vi "Mak Cash Estimator.vi"(10 "Update Stats File?":bool=TRUE, 11 "file path (use dialog)":path=path "C:/Users/manma/Google Drive/WPC Stat Scrape/Data/WPC Stats.bin") -> (0 "Full WPC Stats":T1[][](array[typedef]) {"Date Updated" format="%<%m/%d/%Y>T"}, 1 "Profit/Day":dbl, 2 "Current Value":dbl format="%#_8g", 3 "Cash Profit Over Time":cluster{timestamp[], "Best Linear Fit":dbl[]}[](graph))   [LabVIEW 2021]
uses:
  SubVIs/WPC Player and Financial Stats.ctl
  <vilib>/Analysis/NI_AALPro.lvlib
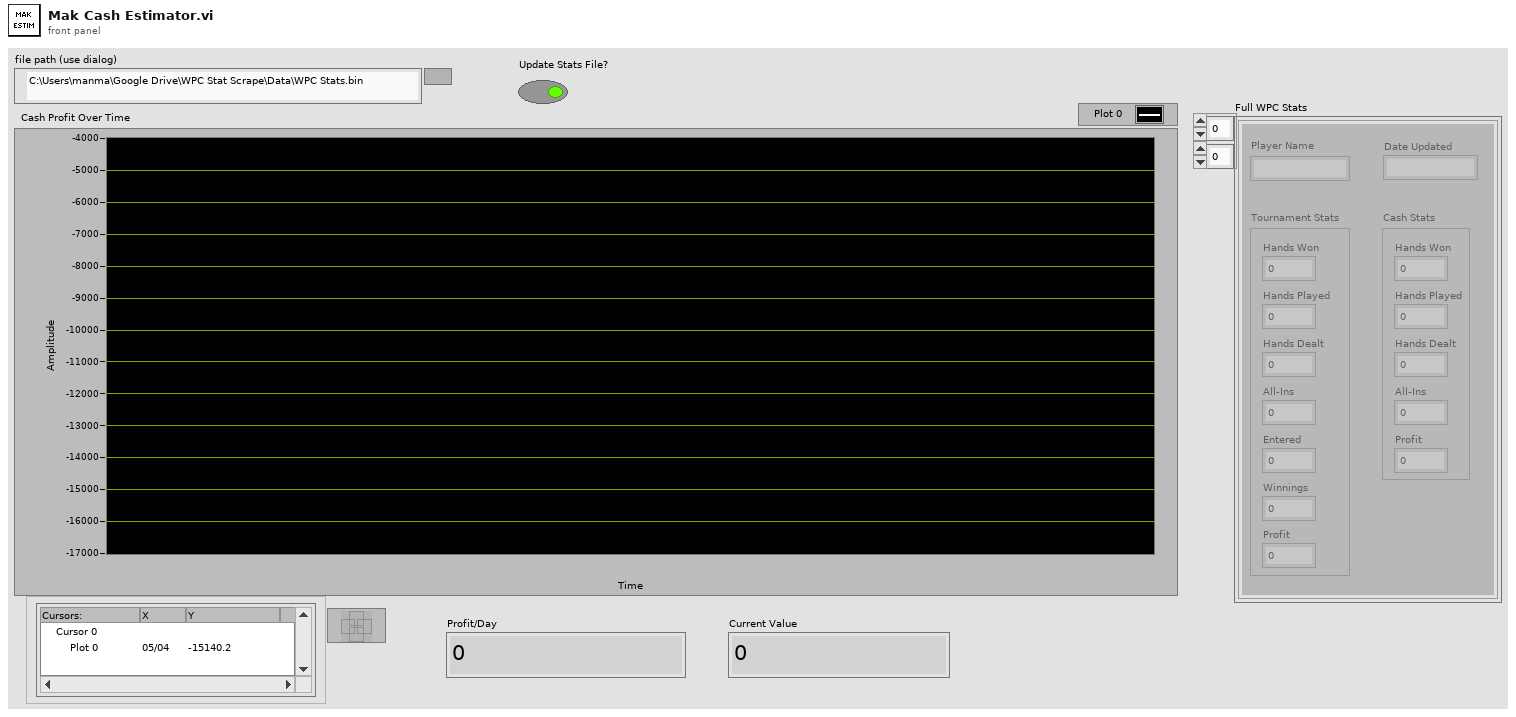
[diagram p1: front panel]
types:
  T1 = typedef "WPC Player and Financial Stats.ctl" = cluster{"Player Name":string, "Date Updated":timestamp, "Tournament Stats":cluster{"Hands Won":i32, "Hands Played":i32, "Hands Dealt":i32, "All-Ins":i32, "Entered":i32, "Winnings":dbl, "Profit":dbl}, "Cash Stats":cluster{"Hands Won":i32, "Hands Played":i32, "Hands Dealt":i32, "All-Ins":i32, "Profit":dbl}}
  T2 = typedef "LVDateTimeRec.ctl" = cluster{"fractional second":dbl, "second":i32, "minute":i32, "hour":i32, "day of month":i32, "month":i32, "year":i32, "day of week":i32, "day of year":i32, "DST":i32}
  T3 = enum16{"open", "replace", "create", "open or create", "replace or create", "replace or create with confirmation"}
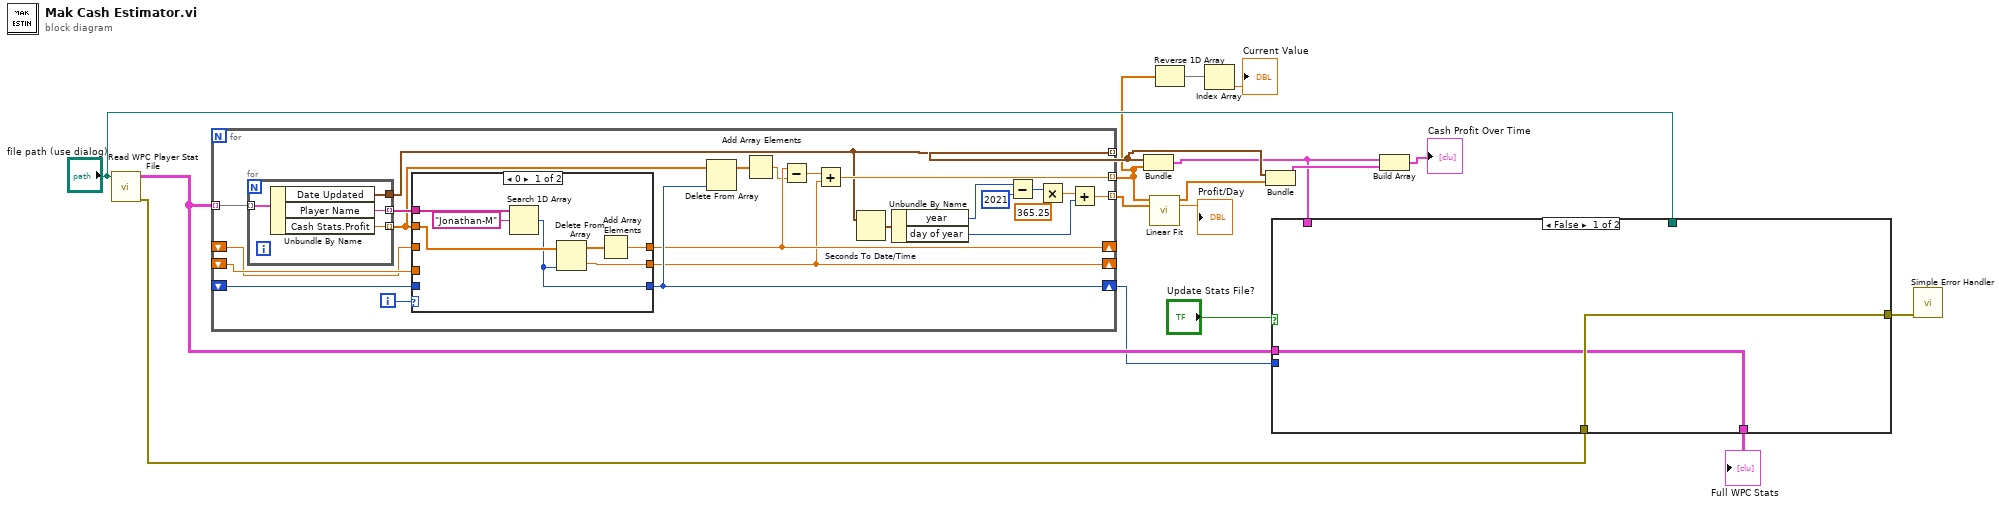
[diagram p0: block diagram]
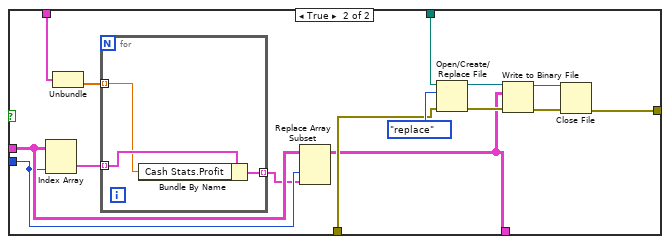
[diagram p2: hidden frame]
diagram:
  n1 = call "Read WPC Player Stat File.vi"("file path (use dialog)"="file path (use dialog)") -> ("error out"=w8:errorcluster, "Full WPC Stats"=w11:T1[][])  [unwired: 8 in, 1 out]
  n2 = for {
    tunnel: w11 -> [w40] mode=indexing
    shift-right: [w29] -> _
    shift-left: _ -> [w35]
    shift-right: [w27] -> _
    shift-left: _ -> [w36]
    shift-right: [w33] -> w10
    shift-left: _ -> [w37]
    tunnel: [w30] -> w4 mode=indexing
    tunnel: [w26] -> w15 mode=indexing
    tunnel: [w18] -> w5 mode=indexing
    i -> [w39]
    n3 = for {
      tunnel: w40 -> [w54] mode=indexing
      tunnel: [w53] -> w26
      tunnel: [w52] -> w38 mode=indexing
      tunnel: [w51] -> w34 mode=indexing
      n4 = Unbundle By Name(w54) -> ("Date Updated"=w53:timestamp, "Player Name"=w52:string, "Cash Stats.Profit"=w51:dbl)
    }
    n5 = case shown="0" w39 {
      tunnel: w38 -> [w47 _]
      tunnel: w34 -> [w45 _]
      tunnel: [w43 w48] -> w29
      tunnel: [w42 w49] -> w27
      tunnel: [w41 w50] -> w33
      tunnel: w37 -> [_ w50]
      tunnel: w36 -> [_ w49]
      tunnel: w35 -> [_ w48]
      frame 0 {
        n6 = Search 1D Array(1D array=w47, element="Jonathan-M") -> (index of element=w41:i32)  [unwired: 1 in]
        n7 = Delete From Array(array=w45, index=w41) -> (deleted portion=w42:dbl, array with subset deleted=w44:dbl[])  [unwired: 1 in]
        n8 = Add Array Elements(numeric array=w44) -> (sum=w43:dbl)
      }
      frame 1.., Default {
      }
    }
    n9 = Delete From Array(array=w34, index=w33) -> (array with subset deleted=w32:dbl[])  [unwired: 1 in, 1 out]
    n10 = Add Array Elements(numeric array=w32) -> (sum=w28:dbl)
    n11 = Subtract(x=w29, y=w28) -> (x-y=w31:dbl)
    n12 = Add(x=w31, y=w27) -> (x+y=w30:dbl)
    n13 = Seconds To Date/Time(time stamp (now)=w26) -> (date time rec=w25:T2)  [unwired: 1 in]
    n14 = Unbundle By Name(w25) -> ("year"=w24:i32, "day of year"=w19:i32)
    n15 = Subtract(x=w24, y=2021) -> (x-y=w22:i32)
    n16 = Multiply(x=w22, y=sgl 365.25) -> (x*y=w20:sgl)
    n17 = Add(x=w20, y=w19) -> (x+y=w18:sgl)
  }
  n18 = Bundle(w15, w4) -> (w9:cluster{timestamp[], dbl[]})  [unwired: 1 in]
  n19 = call <vilib>:"Linear Fit.vi"("Y"=w4, "X"=w5) -> ("Best Linear Fit"=w14:dbl[], "slope"=→"Profit/Day":dbl)  [unwired: 9 in, 3 out]
  n20 = Reverse 1D Array(array=w4) -> (reversed array=w3:dbl[])
  n21 = Index Array(array=w3) -> (element=→"Current Value":dbl)  [unwired: 1 in]
  n22 = Bundle(w15, "Best Linear Fit"=w14) -> (w16:cluster{timestamp[], "Best Linear Fit":dbl[]})  [unwired: 1 in]
  n23 = case shown="False" "Update Stats File?" {
    tunnel: w11 -> [w55 w68]
    tunnel: w10 -> [_ w67]
    tunnel: w9 -> [_ w71]
    tunnel: w8 -> [w56 w60]
    tunnel: "file path (use dialog)" -> [_ w59]
    tunnel: [w56 w58] -> w6
    tunnel: [w55 w57] -> w1
    frame False {
    }
    frame True {
      n24 = Index Array(array=w68, index (col)=w67) -> (element=w70:T1[])  [unwired: 1 in]
      n25 = Unbundle(w71) -> (w69:dbl[])  [unwired: 1 out]
      n26 = for {
        tunnel: w70 -> [w74] mode=indexing
        tunnel: w69 -> [w73] mode=indexing
        tunnel: [w72] -> w66 mode=indexing
        n27 = Bundle By Name(cluster=w74, "Cash Stats.Profit"=w73) -> (w72:T1)
      }
      n28 = Replace Array Subset(array=w68, new element=w66, index (col)=w67) -> (w57:T1[][])  [unwired: 1 in]
      n29 = Open/Create/Replace File(file path (use dialog)=w59, error in=w60, operation (0:open)=T3."replace") -> (refnum out=w63:refnum<file>, error out=w64:errorcluster)  [unwired: 3 in, 1 out]
      n30 = Write to Binary File(file (use dialog)=w63, data=w57, error in=w64) -> (refnum out=w62:refnum<file>, error out=w61:errorcluster)  [unwired: 3 in, 1 out]
      n31 = Close File(refnum=w62, error in=w61) -> (error out=w58:errorcluster)  [unwired: 1 out]
    }
  }
  "Full WPC Stats" <- w1
  n32 = Build Array(w9, w16) -> (→"Cash Profit Over Time":cluster{timestamp[], "Best Linear Fit":dbl[]}[])
  n33 = call <vilib>:"Simple Error Handler.vi"("error in (no error)"=w6) -> ()  [unwired: 4 in, 5 out]
